vi "test_Create FPGA Addon_Error.vi"(8 "error in (no error)":errorcluster, 11 "TestCase in":refnum<class "FPGA Addon Scripting API Unit Tests.lvclass">) -> (0 "error out":errorcluster, 3 "TestCase out":refnum<class "FPGA Addon Scripting API Unit Tests.lvclass">)   [LabVIEW 2021, in "FPGA Addon Scripting API Unit Tests.lvclass"]
uses:
  FPGA Addon Scripting API Unit Tests.lvclass
  <vilib>/addons/_JKI Toolkits/VI Tester/TestCase.llb/TestCase.lvclass
  FPGA Addon Test Class/FPGA Addon Test Class.lvclass
  APIs/Scripting API/Scripting API.lvlib
  C:/Program Files/National Instruments/LabVIEW 2021/vi.lib/addons/_JKI Toolkits/VI Tester/TestCase.llb/TestCase.lvclass
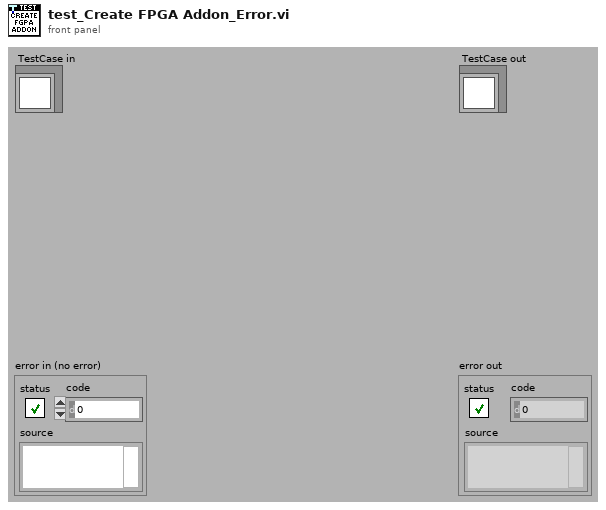
[diagram p1: front panel]
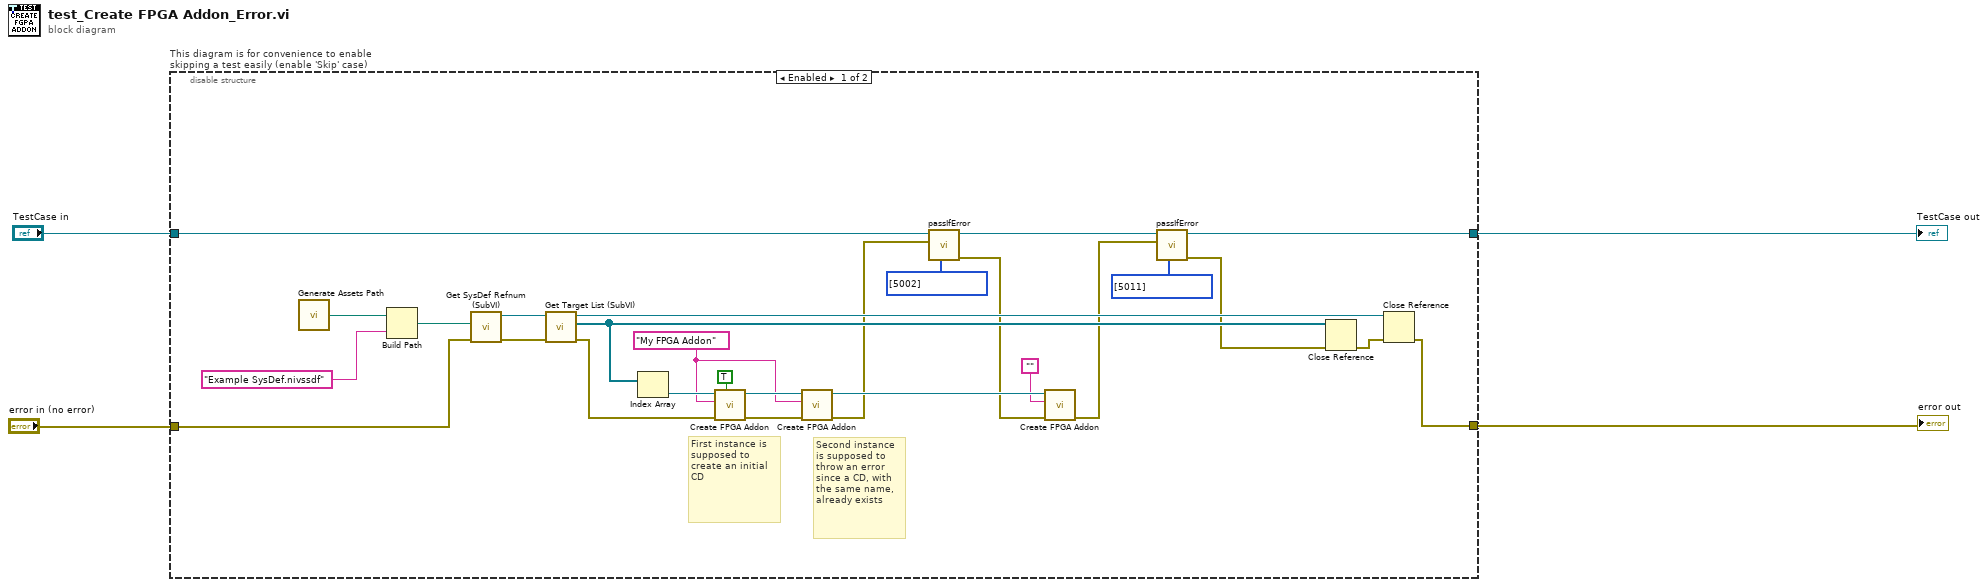
[diagram p0: block diagram]
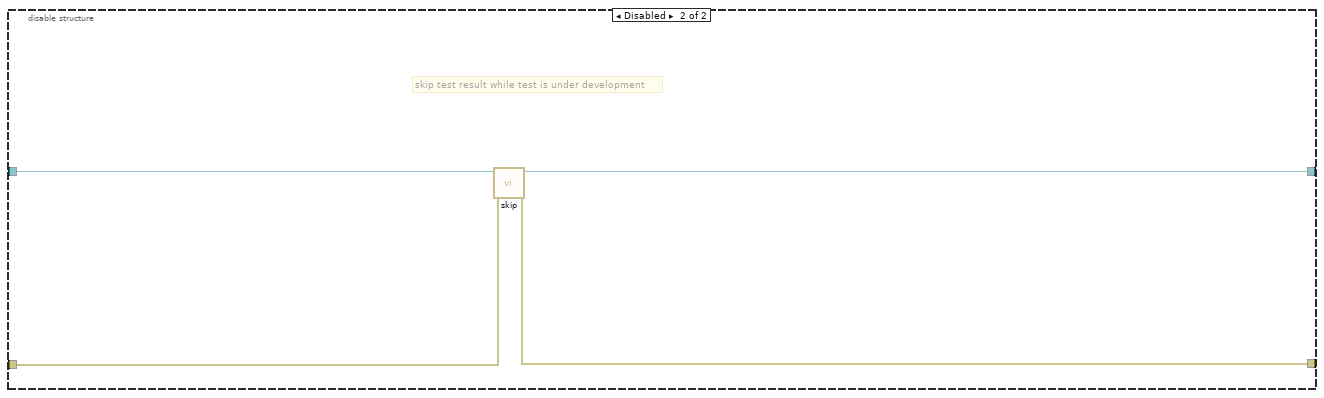
[diagram p2: hidden frame]
diagram:
  n1 = disable-structure "This diagram is for convenience to enable skipping a test easily (enable 'Skip' case)" shown="Enabled" {
    disable-tunnel: "TestCase in" -> [w16 w35]
    disable-tunnel: [w7 w33] -> w1
    disable-tunnel: [w6 w34] -> w3
    disable-tunnel: "error in (no error)" -> [w26 w32]
    frame Enabled {
      w17 = "My FPGA Addon" ("FPGA addon name")
      # "Second instance is supposed to throw an error since a CD, with the same name, already exists"
      # "First instance is supposed to create an initial CD"
      n2 = call "Generate Assets Path.vi"() -> ("Assets path"=w31:path)
      n3 = Build Path(base path=w31, name or relative path="Example SysDef.nivssdf") -> (appended path=w29:path)
      n4 = call "Get SysDef Refnum (SubVI).vi"("error in (no error)"=w26, "System Definition path"=w29) -> ("error out"=w25:errorcluster, "SysDef Refnum out"=w28:refnum<k24>)  [unwired: 8 in]
      n5 = call "Get Target List (SubVI).vi"("error in (no error)"=w25, "SysDef Refnum in"=w28) -> ("error out"=w24:errorcluster, "Target List Refnums"=w23:refnum<k24>[], "SysDef Refnum out"=w22:refnum<k24>)  [unwired: 7 in]
      n6 = Index Array(array=w23) -> (element=w27:refnum<k24>)  [unwired: 1 in]
      n7 = call "Create FPGA Addon.vi"("group scalars"=TRUE, "error in"=w24, "FPGA addon name"=w17, "target in"=w27) -> ("error out"=w19:errorcluster, "target out"=w18:refnum<k24>)  [unwired: 5 in, 1 out]
      n8 = call "Create FPGA Addon.vi"("error in"=w19, "FPGA addon name"=w17, "target in"=w18) -> ("error out"=w11:errorcluster, "target out"=w13:refnum<k24>)  [unwired: 6 in, 1 out]
      n9 = call-dynamic "passIfError.vi"("passing error codes (default = any error code)"=i32[] [5002], "error"=w11, "TestCase in"=w16) -> ("error out"=w10:errorcluster, "TestCase out"=w14:refnum<class "FPGA Addon Scripting API Unit Tests.lvclass">)  [unwired: 7 in]
      n10 = call "Create FPGA Addon.vi"("error in"=w10, "FPGA addon name"="", "target in"=w13) -> ("error out"=w9:errorcluster)  [unwired: 6 in, 2 out]
      n11 = call-dynamic "passIfError.vi"("passing error codes (default = any error code)"=i32[] [5011], "error"=w9, "TestCase in"=w14) -> ("error out"=w5:errorcluster, "TestCase out"=w7:refnum<class "FPGA Addon Scripting API Unit Tests.lvclass">)  [unwired: 7 in]
      n12 = Close Reference(reference=w23, error in (no error)=w5) -> (error out=w21:errorcluster)
      n13 = Close Reference(reference=w22, error in (no error)=w21) -> (error out=w6:errorcluster)
    }
    frame Disabled {
      # "skip test result while test is under development"
      n14 = call <vilib>:"skip.vi"("error in (no error)"=w32, "TestCase in"=w35) -> ("error out"=w34:errorcluster, "TestCase out"=w33:refnum<class "FPGA Addon Scripting API Unit Tests.lvclass">)  [unwired: 8 in]
    }
  }
  "error out" <- w3
  "TestCase out" <- w1
